vi "example-write-read-table.vi"() -> ()   [LabVIEW 2013]
uses:
  cfitsio-hdutypes.ctl
  gfitsio-write-column-u8-scalar.vi
  gfitsio-write-column-u8-1d.vi
  gfitsio-read-column-u8-scalar.vi
  gfitsio-read-column-u8-1d.vi
  gfitsio-write-column-i16-scalar.vi
  gfitsio-write-column-i16-1d.vi
  gfitsio-read-column-i16-scalar.vi
  gfitsio-read-column-i16-1d.vi
  gfitsio-write-column-i32-scalar.vi
  gfitsio-write-column-i32-1d.vi
  gfitsio-read-column-i32-scalar.vi
  gfitsio-read-column-i32-1d.vi
  gfitsio-write-column-sgl-scalar.vi
  gfitsio-write-column-sgl-1d.vi
  gfitsio-read-column-sgl-scalar.vi
  gfitsio-read-column-sgl-1d.vi
  gfitsio-write-column-dbl-scalar.vi
  gfitsio-write-column-dbl-1d.vi
  gfitsio-read-column-dbl-scalar.vi
  gfitsio-read-column-dbl-1d.vi
  gfitsio-write-column-boolean-scalar.vi
  gfitsio-write-column-boolean-1d.vi
  gfitsio-read-column-boolean-scalar.vi
  gfitsio-read-column-boolean-1d.vi
  gfitsio-write-column-csg-scalar.vi
  gfitsio-write-column-csg-1d.vi
  gfitsio-read-column-csg-scalar.vi
  gfitsio-read-column-csg-1d.vi
  gfitsio-write-column-cdb-scalar.vi
  gfitsio-write-column-cdb-1d.vi
  gfitsio-read-column-cdb-scalar.vi
  gfitsio-read-column-cdb-1d.vi
  gfitsio-write-column-string.vi
  gfitsio-read-column-string.vi
  gfitsio-write-column-datetime.vi
  gfitsio-read-column-datetime.vi
  gfitsio.lvlib
panel:
  out "error out":errorcluster
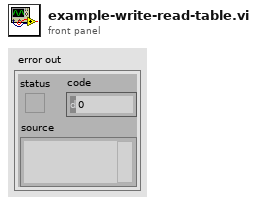
[diagram p1: front panel]
types:
  T1 = enum16{"open", "open or create", "create or replace", "create", "open (read only)"}
  T2 = typedef "gfitsio.lvlib/gfitsio-refnum.ctl" = refnum<k1>
  T3 = typedef "gfitsio.lvlib/cfitsio-hdutypes.ctl" = i32
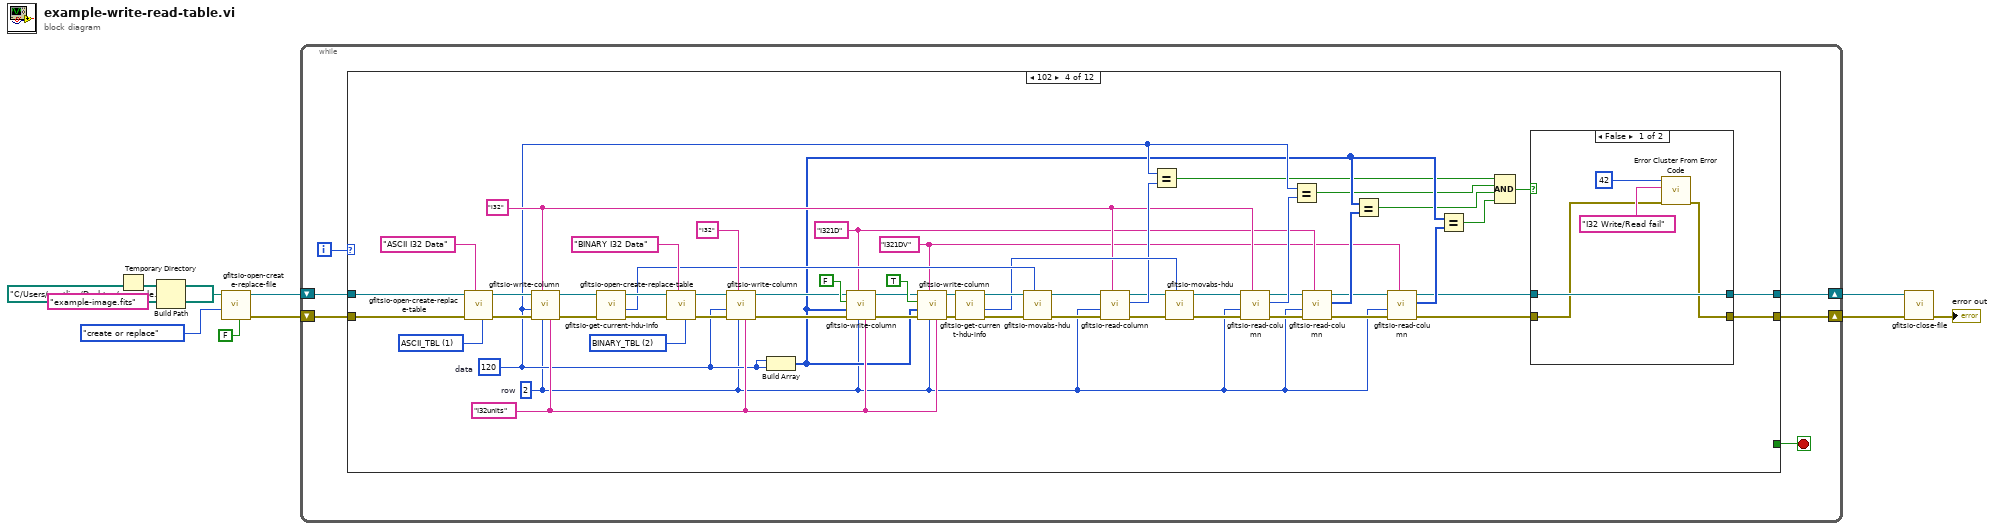
[diagram p0: block diagram]
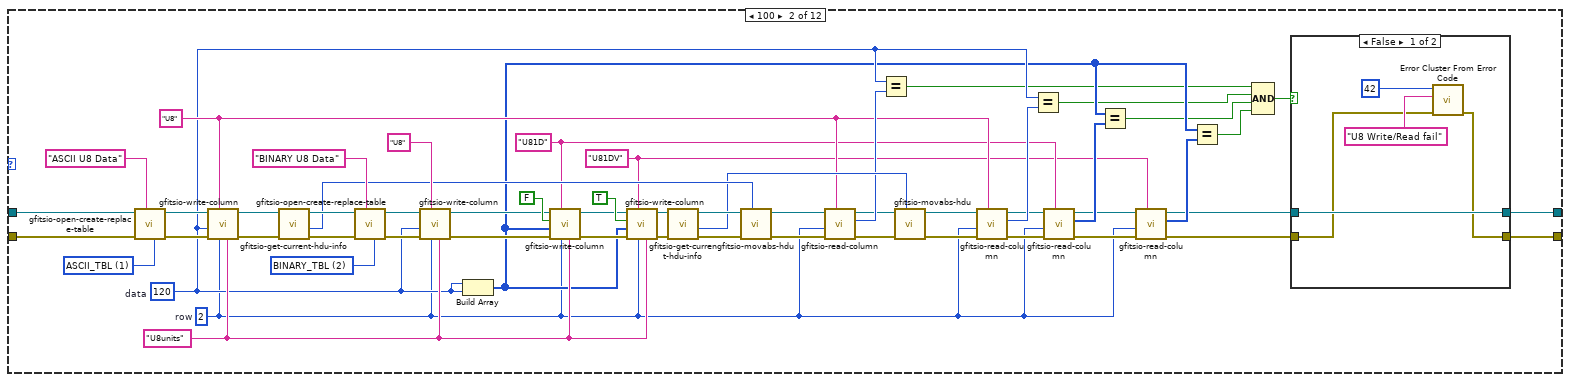
[diagram p3: hidden frame]
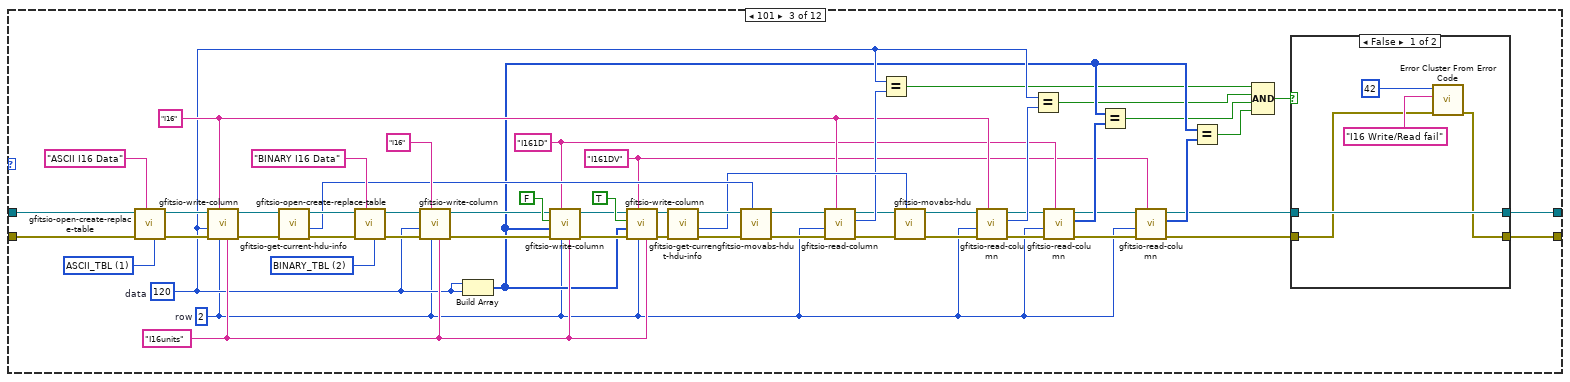
[diagram p5: hidden frame]
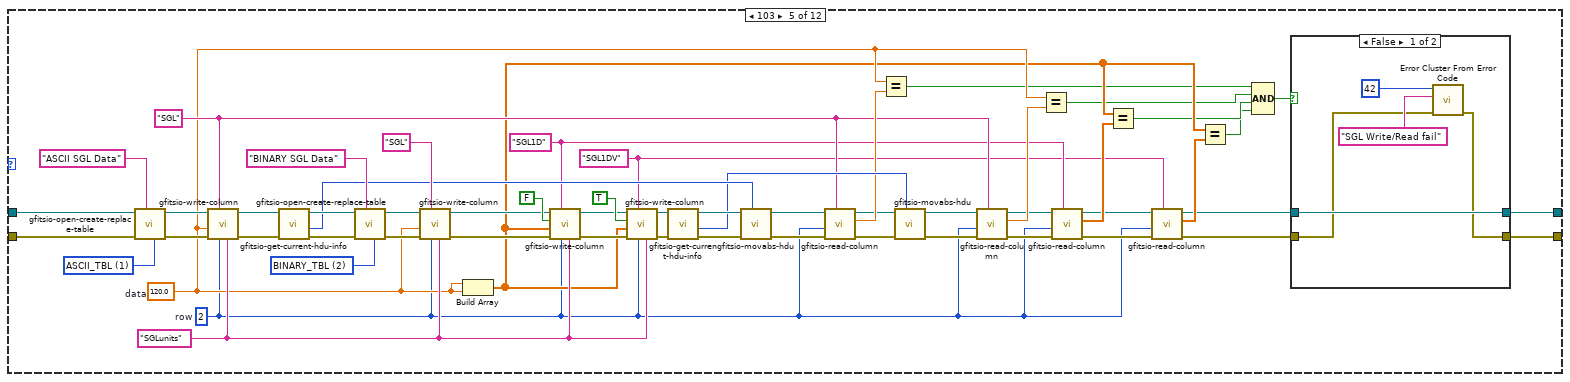
[diagram p8: hidden frame]
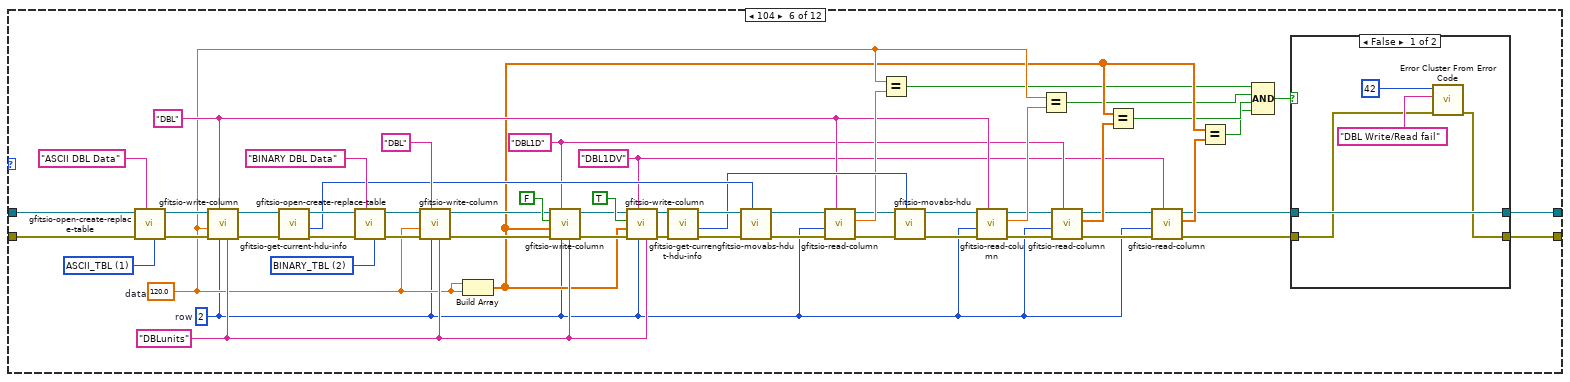
[diagram p10: hidden frame]
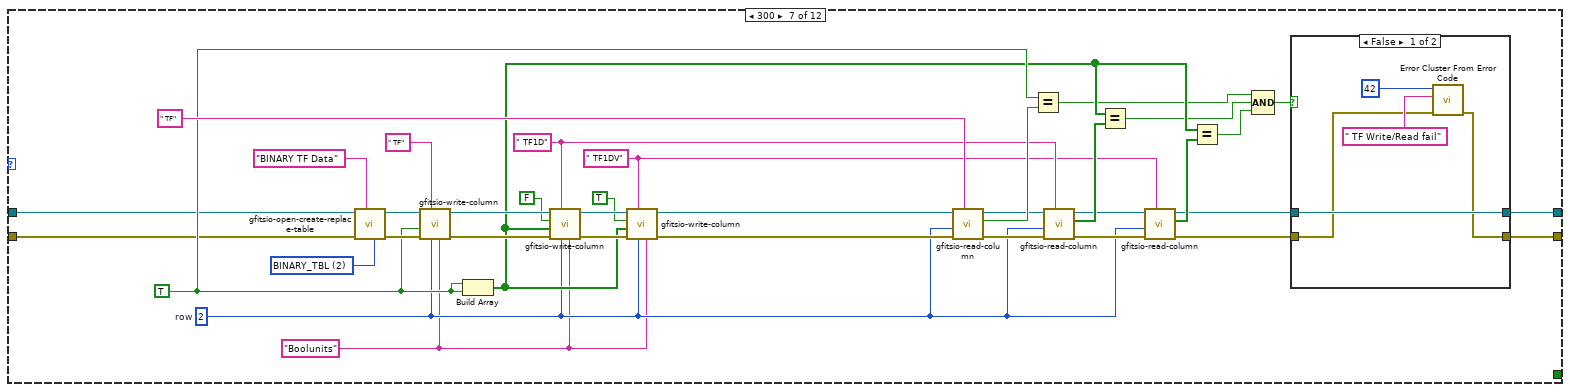
[diagram p12: hidden frame]
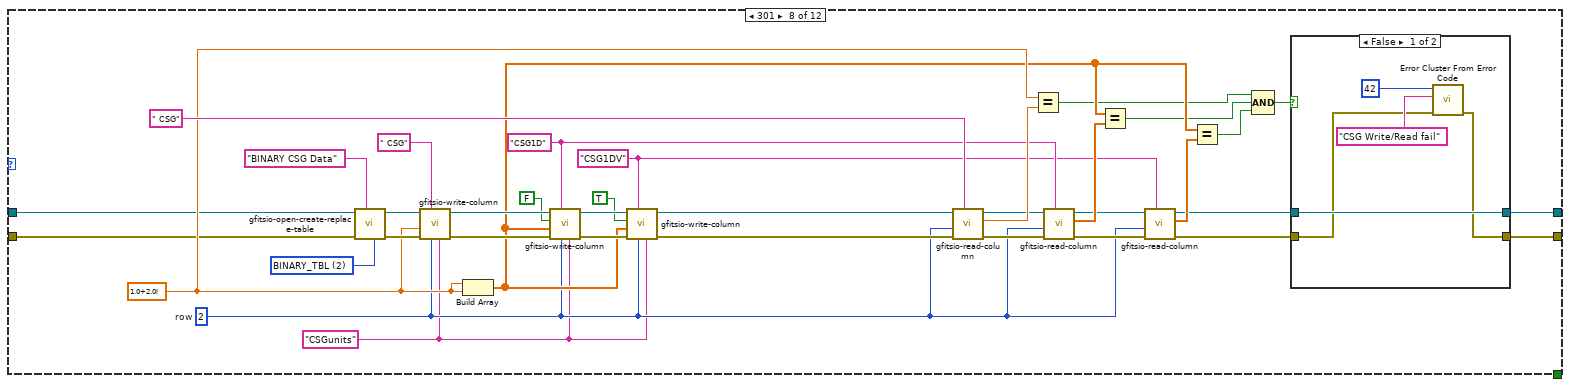
[diagram p14: hidden frame]
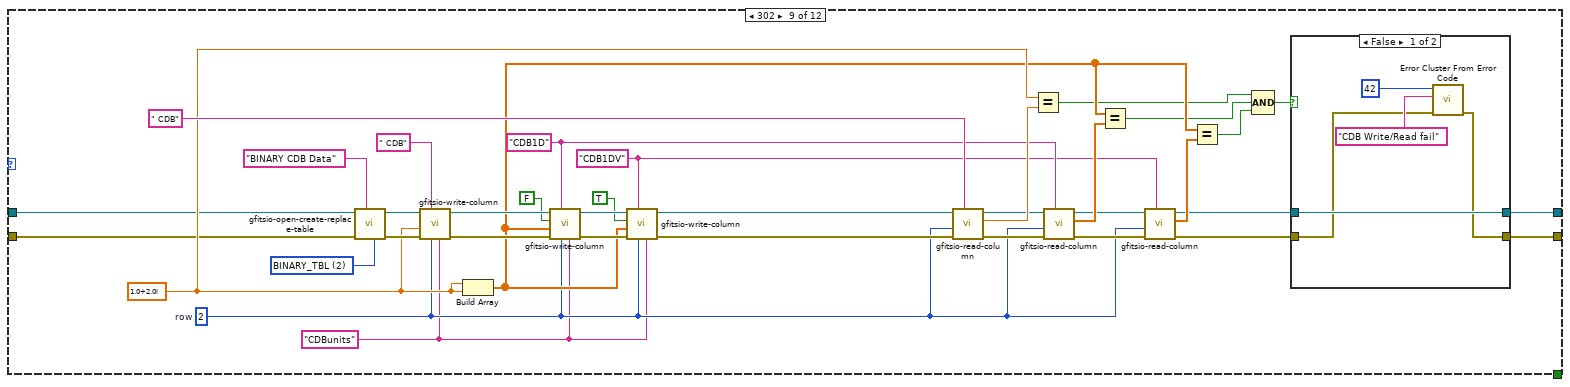
[diagram p16: hidden frame]
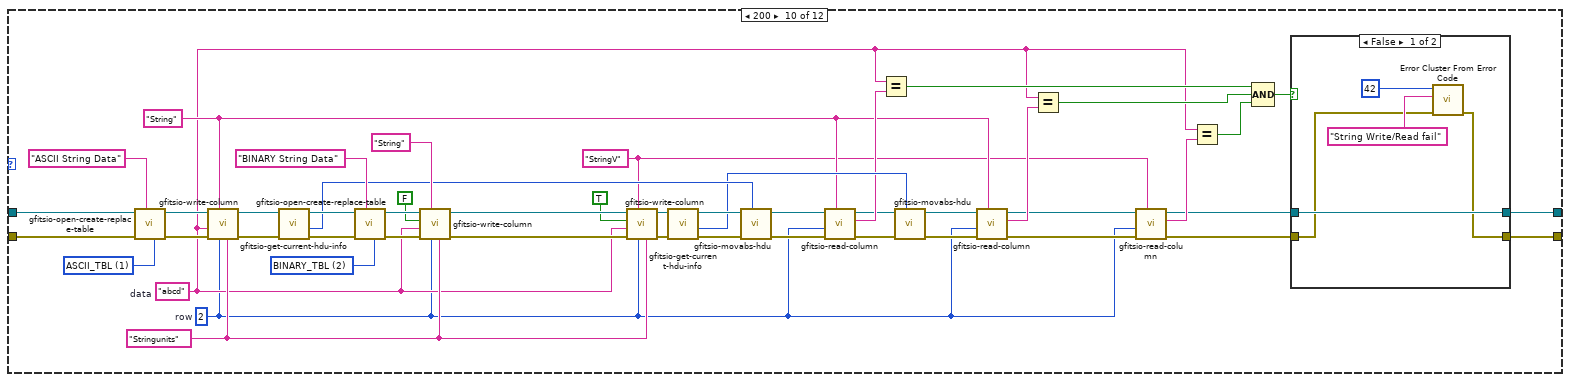
[diagram p18: hidden frame]
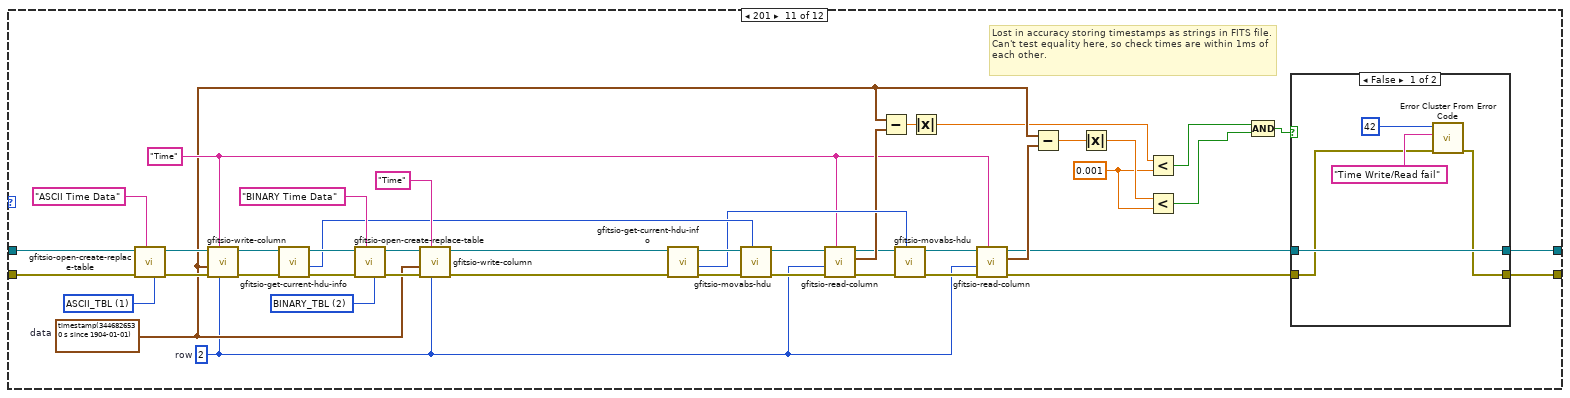
[diagram p20: hidden frame]
diagram:
  n1 = Temporary Directory() -> (w7:path)
  n2 = Build Path(base path=w7, name or relative path="example-image.fits") -> ()  [unwired: 1 out]
  n3 = call "gfitsio-open-create-replace-file.vi"("advisory dialog? (display:T)"=FALSE, "function (open)"=T1."create or replace", "file path (dialog if empty)"=path "C:/Users/ggatling/Desktop/example.fits") -> ("error out"=w9:errorcluster, "gfits refnum"=w10:T2)  [unwired: 6 in, 1 out]
  n4 = while {
    shift-right: [w14] -> w2
    shift-left: w10 -> [w16]
    shift-right: [w13] -> w1
    shift-left: w9 -> [w15]
    i -> [w12]
    stop <- w11 stop-if-true
    n5 = case shown="102" w12 {
      tunnel: w16 -> [w18 w75 w139 w203 w267 w331 w346 w390 w434 w519 w570 w580]
      tunnel: w15 -> [w17 w74 w138 w202 w266 w330 w345 w389 w433 w518 w569 w579]
      tunnel: [w18 w21 w85 w149 w213 w277 w348 w392 w436 w476 w539 w580] -> w14
      tunnel: [w17 w20 w84 w148 w212 w276 w347 w391 w435 w475 w538 w579] -> w13
      tunnel: [_ _ _ _ _ _ _ _ _ _ _ TRUE] -> w11
      frame Default {
      }
      frame 100 {
        w69 = T3 2 items=["ANY_HDU"=-1, "IMAGE_HDU"=0, "ASCII_TBL"=1, "BINARY_TBL"=2] ("table type (binary)")
        w33 = "U81DV" ("column")
        w34 = "U81D" ("column")
        w70 = T3 1 items=["ANY_HDU"=-1, "IMAGE_HDU"=0, "ASCII_TBL"=1, "BINARY_TBL"=2] ("table type (binary)")
        w58 = "U8units" ("units")
        w19 = 2  # row
        w30 = u8 120  # data
        w36 = "U8" ("column")
        n6 = call "gfitsio-open-create-replace-table.vi"("table type (binary)"=w70, "hdu name (dialog if empty)"="ASCII U8 Data", "error in (no error)"=w74, "gfits refnum"=w75) -> ("error out"=w72:errorcluster, "dup gfits refnum"=w73:T2)  [unwired: 5 in, 1 out]
        n7 = call-poly "gfitsio-write-column.vi"("units"=w58, "row"=w19, "column"=w36, "error in (no error)"=w72, "data"=w30, "gfits refnum"=w73) -> ("error out"=w56:errorcluster, "dup gfits refnum"=w57:T2)  [unwired: 4 in]
        n8 = call "gfitsio-get-current-hdu-info.vi"("error in (no error)"=w56, "gfits refnum"=w57) -> ("error out"=w51:errorcluster, "hdu number"=w49:i32, "dup gfits refnum"=w50:T2)  [unwired: 5 in, 2 out]
        n9 = call "gfitsio-open-create-replace-table.vi"("table type (binary)"=w69, "hdu name (dialog if empty)"="BINARY U8 Data", "error in (no error)"=w51, "gfits refnum"=w50) -> ("error out"=w60:errorcluster, "dup gfits refnum"=w59:T2)  [unwired: 5 in, 1 out]
        n10 = call-poly "gfitsio-write-column.vi"("units"=w58, "row"=w19, "column"="U8", "error in (no error)"=w60, "data"=w30, "gfits refnum"=w59) -> ("error out"=w64:errorcluster, "dup gfits refnum"=w63:T2)  [unwired: 4 in]
        n11 = Build Array(w30, w30) -> (w29:u8[])
        n12 = call-poly "gfitsio-write-column.vi"("units"=w58, "row"=w19, "column"=w34, "error in (no error)"=w64, "data"=w29, "variable length? (T:yes)"=FALSE, "gfits refnum"=w63) -> ("error out"=w66:errorcluster, "dup gfits refnum"=w65:T2)  [unwired: 3 in]
        n13 = call-poly "gfitsio-write-column.vi"("units"=w58, "row"=w19, "column"=w33, "error in (no error)"=w66, "data"=w29, "variable length? (T:yes)"=TRUE, "gfits refnum"=w65) -> ("error out"=w55:errorcluster, "dup gfits refnum"=w54:T2)  [unwired: 3 in]
        n14 = call "gfitsio-get-current-hdu-info.vi"("error in (no error)"=w55, "gfits refnum"=w54) -> ("error out"=w53:errorcluster, "hdu number"=w48:i32, "dup gfits refnum"=w52:T2)  [unwired: 5 in, 2 out]
        n15 = call "gfitsio-movabs-hdu.vi"("hdunum"=w49, "error in (no error)"=w53, "gfits refnum"=w52) -> ("error out"=w46:errorcluster, "dup gfits refnum"=w47:T2)  [unwired: 6 in, 1 out]
        n16 = call-poly "gfitsio-read-column.vi"("column"=w36, "error in (no error)"=w46, "row"=w19, "gfits refnum"=w47) -> ("error out"=w41:errorcluster, "data"=w45:u8, "dup gfits refnum"=w42:T2)  [unwired: 5 in]
        n17 = Equal?(x=w30, y=w45) -> (x = y?=w28:bool)
        n18 = call "gfitsio-movabs-hdu.vi"("hdunum"=w48, "error in (no error)"=w41, "gfits refnum"=w42) -> ("error out"=w39:errorcluster, "dup gfits refnum"=w40:T2)  [unwired: 6 in, 1 out]
        n19 = call-poly "gfitsio-read-column.vi"("column"=w36, "error in (no error)"=w39, "row"=w19, "gfits refnum"=w40) -> ("error out"=w37:errorcluster, "data"=w44:u8, "dup gfits refnum"=w38:T2)  [unwired: 5 in]
        n20 = Equal?(x=w30, y=w44) -> (x = y?=w27:bool)
        n21 = call-poly "gfitsio-read-column.vi"("column"=w34, "error in (no error)"=w37, "row"=w19, "gfits refnum"=w38) -> ("error out"=w31:errorcluster, "data"=w43:u8[], "dup gfits refnum"=w32:T2)  [unwired: 5 in]
        n22 = Equal?(x=w29, y=w43) -> (x = y?=w26:bool)
        n23 = call-poly "gfitsio-read-column.vi"("column"=w33, "error in (no error)"=w31, "row"=w19, "gfits refnum"=w32) -> ("error out"=w23:errorcluster, "data"=w35:u8[], "dup gfits refnum"=w24:T2)  [unwired: 5 in]
        n24 = Equal?(x=w29, y=w35) -> (x = y?=w25:bool)
        n25 = Compound Arithmetic op=AND(w28, w27, w26, w25) -> (w22:bool)
        n26 = case shown="False" w22 {
          tunnel: w24 -> [w80 w82]
          tunnel: w23 -> [w77 w81]
          tunnel: [w80 w82] -> w21
          tunnel: [w76 w81] -> w20
          frame False {
            n27 = call <vilib>:"Error Cluster From Error Code.vi"("error in (no error)"=w77, "error message (\"\")"="U8 Write/Read fail" ("error message (\"\")"), "error code (0)"=42) -> ("error out"=w76:errorcluster)  [unwired: 6 in]
          }
          frame True {
          }
        }
      }
      frame 101 {
        w133 = T3 2 items=["ANY_HDU"=-1, "IMAGE_HDU"=0, "ASCII_TBL"=1, "BINARY_TBL"=2] ("table type (binary)")
        w97 = "I161DV" ("column")
        w98 = "I161D" ("column")
        w134 = T3 1 items=["ANY_HDU"=-1, "IMAGE_HDU"=0, "ASCII_TBL"=1, "BINARY_TBL"=2] ("table type (binary)")
        w122 = "I16units" ("units")
        w83 = 2  # row
        w94 = i16 120  # data
        w100 = "I16" ("column")
        n28 = call "gfitsio-open-create-replace-table.vi"("table type (binary)"=w134, "hdu name (dialog if empty)"="ASCII I16 Data", "error in (no error)"=w138, "gfits refnum"=w139) -> ("error out"=w136:errorcluster, "dup gfits refnum"=w137:T2)  [unwired: 5 in, 1 out]
        n29 = call-poly "gfitsio-write-column.vi"("units"=w122, "row"=w83, "column"=w100, "error in (no error)"=w136, "data"=w94, "gfits refnum"=w137) -> ("error out"=w120:errorcluster, "dup gfits refnum"=w121:T2)  [unwired: 4 in]
        n30 = call "gfitsio-get-current-hdu-info.vi"("error in (no error)"=w120, "gfits refnum"=w121) -> ("error out"=w115:errorcluster, "hdu number"=w113:i32, "dup gfits refnum"=w114:T2)  [unwired: 5 in, 2 out]
        n31 = call "gfitsio-open-create-replace-table.vi"("table type (binary)"=w133, "hdu name (dialog if empty)"="BINARY I16 Data", "error in (no error)"=w115, "gfits refnum"=w114) -> ("error out"=w124:errorcluster, "dup gfits refnum"=w123:T2)  [unwired: 5 in, 1 out]
        n32 = call-poly "gfitsio-write-column.vi"("units"=w122, "row"=w83, "column"="I16", "error in (no error)"=w124, "data"=w94, "gfits refnum"=w123) -> ("error out"=w128:errorcluster, "dup gfits refnum"=w127:T2)  [unwired: 4 in]
        n33 = Build Array(w94, w94) -> (w93:i16[])
        n34 = call-poly "gfitsio-write-column.vi"("units"=w122, "row"=w83, "column"=w98, "error in (no error)"=w128, "data"=w93, "variable length? (T:yes)"=FALSE, "gfits refnum"=w127) -> ("error out"=w130:errorcluster, "dup gfits refnum"=w129:T2)  [unwired: 3 in]
        n35 = call-poly "gfitsio-write-column.vi"("units"=w122, "row"=w83, "column"=w97, "error in (no error)"=w130, "data"=w93, "variable length? (T:yes)"=TRUE, "gfits refnum"=w129) -> ("error out"=w119:errorcluster, "dup gfits refnum"=w118:T2)  [unwired: 3 in]
        n36 = call "gfitsio-get-current-hdu-info.vi"("error in (no error)"=w119, "gfits refnum"=w118) -> ("error out"=w117:errorcluster, "hdu number"=w112:i32, "dup gfits refnum"=w116:T2)  [unwired: 5 in, 2 out]
        n37 = call "gfitsio-movabs-hdu.vi"("hdunum"=w113, "error in (no error)"=w117, "gfits refnum"=w116) -> ("error out"=w110:errorcluster, "dup gfits refnum"=w111:T2)  [unwired: 6 in, 1 out]
        n38 = call-poly "gfitsio-read-column.vi"("column"=w100, "error in (no error)"=w110, "row"=w83, "gfits refnum"=w111) -> ("error out"=w105:errorcluster, "data"=w109:i16, "dup gfits refnum"=w106:T2)  [unwired: 5 in]
        n39 = Equal?(x=w94, y=w109) -> (x = y?=w92:bool)
        n40 = call "gfitsio-movabs-hdu.vi"("hdunum"=w112, "error in (no error)"=w105, "gfits refnum"=w106) -> ("error out"=w103:errorcluster, "dup gfits refnum"=w104:T2)  [unwired: 6 in, 1 out]
        n41 = call-poly "gfitsio-read-column.vi"("column"=w100, "error in (no error)"=w103, "row"=w83, "gfits refnum"=w104) -> ("error out"=w101:errorcluster, "data"=w108:i16, "dup gfits refnum"=w102:T2)  [unwired: 5 in]
        n42 = Equal?(x=w94, y=w108) -> (x = y?=w91:bool)
        n43 = call-poly "gfitsio-read-column.vi"("column"=w98, "error in (no error)"=w101, "row"=w83, "gfits refnum"=w102) -> ("error out"=w95:errorcluster, "data"=w107:i16[], "dup gfits refnum"=w96:T2)  [unwired: 5 in]
        n44 = Equal?(x=w93, y=w107) -> (x = y?=w90:bool)
        n45 = call-poly "gfitsio-read-column.vi"("column"=w97, "error in (no error)"=w95, "row"=w83, "gfits refnum"=w96) -> ("error out"=w87:errorcluster, "data"=w99:i16[], "dup gfits refnum"=w88:T2)  [unwired: 5 in]
        n46 = Equal?(x=w93, y=w99) -> (x = y?=w89:bool)
        n47 = Compound Arithmetic op=AND(w92, w91, w90, w89) -> (w86:bool)
        n48 = case shown="False" w86 {
          tunnel: w88 -> [w144 w146]
          tunnel: w87 -> [w141 w145]
          tunnel: [w144 w146] -> w85
          tunnel: [w140 w145] -> w84
          frame False {
            n49 = call <vilib>:"Error Cluster From Error Code.vi"("error in (no error)"=w141, "error message (\"\")"="I16 Write/Read fail" ("error message (\"\")"), "error code (0)"=42) -> ("error out"=w140:errorcluster)  [unwired: 6 in]
          }
          frame True {
          }
        }
      }
      frame 102 {
        w197 = T3 2 items=["ANY_HDU"=-1, "IMAGE_HDU"=0, "ASCII_TBL"=1, "BINARY_TBL"=2] ("table type (binary)")
        w161 = "I321DV" ("column")
        w162 = "I321D" ("column")
        w198 = T3 1 items=["ANY_HDU"=-1, "IMAGE_HDU"=0, "ASCII_TBL"=1, "BINARY_TBL"=2] ("table type (binary)")
        w186 = "I32units" ("units")
        w147 = 2  # row
        w158 = 120  # data
        w164 = "I32" ("column")
        n50 = call "gfitsio-open-create-replace-table.vi"("table type (binary)"=w198, "hdu name (dialog if empty)"="ASCII I32 Data", "error in (no error)"=w202, "gfits refnum"=w203) -> ("error out"=w200:errorcluster, "dup gfits refnum"=w201:T2)  [unwired: 5 in, 1 out]
        n51 = call-poly "gfitsio-write-column.vi"("units"=w186, "row"=w147, "column"=w164, "error in (no error)"=w200, "data"=w158, "gfits refnum"=w201) -> ("error out"=w184:errorcluster, "dup gfits refnum"=w185:T2)  [unwired: 4 in]
        n52 = call "gfitsio-get-current-hdu-info.vi"("error in (no error)"=w184, "gfits refnum"=w185) -> ("error out"=w179:errorcluster, "hdu number"=w177:i32, "dup gfits refnum"=w178:T2)  [unwired: 5 in, 2 out]
        n53 = call "gfitsio-open-create-replace-table.vi"("table type (binary)"=w197, "hdu name (dialog if empty)"="BINARY I32 Data", "error in (no error)"=w179, "gfits refnum"=w178) -> ("error out"=w188:errorcluster, "dup gfits refnum"=w187:T2)  [unwired: 5 in, 1 out]
        n54 = call-poly "gfitsio-write-column.vi"("units"=w186, "row"=w147, "column"="I32", "error in (no error)"=w188, "data"=w158, "gfits refnum"=w187) -> ("error out"=w192:errorcluster, "dup gfits refnum"=w191:T2)  [unwired: 4 in]
        n55 = Build Array(w158, w158) -> (w157:i32[])
        n56 = call-poly "gfitsio-write-column.vi"("units"=w186, "row"=w147, "column"=w162, "error in (no error)"=w192, "data"=w157, "variable length? (T:yes)"=FALSE, "gfits refnum"=w191) -> ("error out"=w194:errorcluster, "dup gfits refnum"=w193:T2)  [unwired: 3 in]
        n57 = call-poly "gfitsio-write-column.vi"("units"=w186, "row"=w147, "column"=w161, "error in (no error)"=w194, "data"=w157, "variable length? (T:yes)"=TRUE, "gfits refnum"=w193) -> ("error out"=w183:errorcluster, "dup gfits refnum"=w182:T2)  [unwired: 3 in]
        n58 = call "gfitsio-get-current-hdu-info.vi"("error in (no error)"=w183, "gfits refnum"=w182) -> ("error out"=w181:errorcluster, "hdu number"=w176:i32, "dup gfits refnum"=w180:T2)  [unwired: 5 in, 2 out]
        n59 = call "gfitsio-movabs-hdu.vi"("hdunum"=w177, "error in (no error)"=w181, "gfits refnum"=w180) -> ("error out"=w174:errorcluster, "dup gfits refnum"=w175:T2)  [unwired: 6 in, 1 out]
        n60 = call-poly "gfitsio-read-column.vi"("column"=w164, "error in (no error)"=w174, "row"=w147, "gfits refnum"=w175) -> ("error out"=w169:errorcluster, "data"=w173:i32, "dup gfits refnum"=w170:T2)  [unwired: 5 in]
        n61 = Equal?(x=w158, y=w173) -> (x = y?=w156:bool)
        n62 = call "gfitsio-movabs-hdu.vi"("hdunum"=w176, "error in (no error)"=w169, "gfits refnum"=w170) -> ("error out"=w167:errorcluster, "dup gfits refnum"=w168:T2)  [unwired: 6 in, 1 out]
        n63 = call-poly "gfitsio-read-column.vi"("column"=w164, "error in (no error)"=w167, "row"=w147, "gfits refnum"=w168) -> ("error out"=w165:errorcluster, "data"=w172:i32, "dup gfits refnum"=w166:T2)  [unwired: 5 in]
        n64 = Equal?(x=w158, y=w172) -> (x = y?=w155:bool)
        n65 = call-poly "gfitsio-read-column.vi"("column"=w162, "error in (no error)"=w165, "row"=w147, "gfits refnum"=w166) -> ("error out"=w159:errorcluster, "data"=w171:i32[], "dup gfits refnum"=w160:T2)  [unwired: 5 in]
        n66 = Equal?(x=w157, y=w171) -> (x = y?=w154:bool)
        n67 = call-poly "gfitsio-read-column.vi"("column"=w161, "error in (no error)"=w159, "row"=w147, "gfits refnum"=w160) -> ("error out"=w151:errorcluster, "data"=w163:i32[], "dup gfits refnum"=w152:T2)  [unwired: 5 in]
        n68 = Equal?(x=w157, y=w163) -> (x = y?=w153:bool)
        n69 = Compound Arithmetic op=AND(w156, w155, w154, w153) -> (w150:bool)
        n70 = case shown="False" w150 {
          tunnel: w152 -> [w208 w210]
          tunnel: w151 -> [w205 w209]
          tunnel: [w208 w210] -> w149
          tunnel: [w204 w209] -> w148
          frame False {
            n71 = call <vilib>:"Error Cluster From Error Code.vi"("error in (no error)"=w205, "error message (\"\")"="I32 Write/Read fail" ("error message (\"\")"), "error code (0)"=42) -> ("error out"=w204:errorcluster)  [unwired: 6 in]
          }
          frame True {
          }
        }
      }
      frame 103 {
        w261 = T3 2 items=["ANY_HDU"=-1, "IMAGE_HDU"=0, "ASCII_TBL"=1, "BINARY_TBL"=2] ("table type (binary)")
        w225 = "SGL1DV" ("column")
        w226 = "SGL1D" ("column")
        w262 = T3 1 items=["ANY_HDU"=-1, "IMAGE_HDU"=0, "ASCII_TBL"=1, "BINARY_TBL"=2] ("table type (binary)")
        w250 = "SGLunits" ("units")
        w211 = 2  # row
        w222 = sgl 120.0  # data
        w228 = "SGL" ("column")
        n72 = call "gfitsio-open-create-replace-table.vi"("table type (binary)"=w262, "hdu name (dialog if empty)"="ASCII SGL Data", "error in (no error)"=w266, "gfits refnum"=w267) -> ("error out"=w264:errorcluster, "dup gfits refnum"=w265:T2)  [unwired: 5 in, 1 out]
        n73 = call-poly "gfitsio-write-column.vi"("units"=w250, "row"=w211, "column"=w228, "error in (no error)"=w264, "data"=w222, "gfits refnum"=w265) -> ("error out"=w248:errorcluster, "dup gfits refnum"=w249:T2)  [unwired: 4 in]
        n74 = call "gfitsio-get-current-hdu-info.vi"("error in (no error)"=w248, "gfits refnum"=w249) -> ("error out"=w243:errorcluster, "hdu number"=w241:i32, "dup gfits refnum"=w242:T2)  [unwired: 5 in, 2 out]
        n75 = call "gfitsio-open-create-replace-table.vi"("table type (binary)"=w261, "hdu name (dialog if empty)"="BINARY SGL Data", "error in (no error)"=w243, "gfits refnum"=w242) -> ("error out"=w252:errorcluster, "dup gfits refnum"=w251:T2)  [unwired: 5 in, 1 out]
        n76 = call-poly "gfitsio-write-column.vi"("units"=w250, "row"=w211, "column"="SGL", "error in (no error)"=w252, "data"=w222, "gfits refnum"=w251) -> ("error out"=w256:errorcluster, "dup gfits refnum"=w255:T2)  [unwired: 4 in]
        n77 = Build Array(w222, w222) -> (w221:sgl[])
        n78 = call-poly "gfitsio-write-column.vi"("units"=w250, "row"=w211, "column"=w226, "error in (no error)"=w256, "data"=w221, "variable length? (T:yes)"=FALSE, "gfits refnum"=w255) -> ("error out"=w258:errorcluster, "dup gfits refnum"=w257:T2)  [unwired: 3 in]
        n79 = call-poly "gfitsio-write-column.vi"("units"=w250, "row"=w211, "column"=w225, "error in (no error)"=w258, "data"=w221, "variable length? (T:yes)"=TRUE, "gfits refnum"=w257) -> ("error out"=w247:errorcluster, "dup gfits refnum"=w246:T2)  [unwired: 3 in]
        n80 = call "gfitsio-get-current-hdu-info.vi"("error in (no error)"=w247, "gfits refnum"=w246) -> ("error out"=w245:errorcluster, "hdu number"=w240:i32, "dup gfits refnum"=w244:T2)  [unwired: 5 in, 2 out]
        n81 = call "gfitsio-movabs-hdu.vi"("hdunum"=w241, "error in (no error)"=w245, "gfits refnum"=w244) -> ("error out"=w238:errorcluster, "dup gfits refnum"=w239:T2)  [unwired: 6 in, 1 out]
        n82 = call-poly "gfitsio-read-column.vi"("column"=w228, "error in (no error)"=w238, "row"=w211, "gfits refnum"=w239) -> ("error out"=w233:errorcluster, "data"=w237:sgl, "dup gfits refnum"=w234:T2)  [unwired: 5 in]
        n83 = Equal?(x=w222, y=w237) -> (x = y?=w220:bool)
        n84 = call "gfitsio-movabs-hdu.vi"("hdunum"=w240, "error in (no error)"=w233, "gfits refnum"=w234) -> ("error out"=w231:errorcluster, "dup gfits refnum"=w232:T2)  [unwired: 6 in, 1 out]
        n85 = call-poly "gfitsio-read-column.vi"("column"=w228, "error in (no error)"=w231, "row"=w211, "gfits refnum"=w232) -> ("error out"=w229:errorcluster, "data"=w236:sgl, "dup gfits refnum"=w230:T2)  [unwired: 5 in]
        n86 = Equal?(x=w222, y=w236) -> (x = y?=w219:bool)
        n87 = call-poly "gfitsio-read-column.vi"("column"=w226, "error in (no error)"=w229, "row"=w211, "gfits refnum"=w230) -> ("error out"=w223:errorcluster, "data"=w235:sgl[], "dup gfits refnum"=w224:T2)  [unwired: 5 in]
        n88 = Equal?(x=w221, y=w235) -> (x = y?=w218:bool)
        n89 = call-poly "gfitsio-read-column.vi"("column"=w225, "error in (no error)"=w223, "row"=w211, "gfits refnum"=w224) -> ("error out"=w215:errorcluster, "data"=w227:sgl[], "dup gfits refnum"=w216:T2)  [unwired: 5 in]
        n90 = Equal?(x=w221, y=w227) -> (x = y?=w217:bool)
        n91 = Compound Arithmetic op=AND(w220, w219, w218, w217) -> (w214:bool)
        n92 = case shown="False" w214 {
          tunnel: w216 -> [w272 w274]
          tunnel: w215 -> [w269 w273]
          tunnel: [w272 w274] -> w213
          tunnel: [w268 w273] -> w212
          frame False {
            n93 = call <vilib>:"Error Cluster From Error Code.vi"("error in (no error)"=w269, "error message (\"\")"="SGL Write/Read fail" ("error message (\"\")"), "error code (0)"=42) -> ("error out"=w268:errorcluster)  [unwired: 6 in]
          }
          frame True {
          }
        }
      }
      frame 104 {
        w325 = T3 2 items=["ANY_HDU"=-1, "IMAGE_HDU"=0, "ASCII_TBL"=1, "BINARY_TBL"=2] ("table type (binary)")
        w289 = "DBL1DV" ("column")
        w290 = "DBL1D" ("column")
        w326 = T3 1 items=["ANY_HDU"=-1, "IMAGE_HDU"=0, "ASCII_TBL"=1, "BINARY_TBL"=2] ("table type (binary)")
        w314 = "DBLunits" ("units")
        w275 = 2  # row
        w286 = 120.0  # data
        w292 = "DBL" ("column")
        n94 = call "gfitsio-open-create-replace-table.vi"("table type (binary)"=w326, "hdu name (dialog if empty)"="ASCII DBL Data", "error in (no error)"=w330, "gfits refnum"=w331) -> ("error out"=w328:errorcluster, "dup gfits refnum"=w329:T2)  [unwired: 5 in, 1 out]
        n95 = call-poly "gfitsio-write-column.vi"("units"=w314, "row"=w275, "column"=w292, "error in (no error)"=w328, "data"=w286, "gfits refnum"=w329) -> ("error out"=w312:errorcluster, "dup gfits refnum"=w313:T2)  [unwired: 4 in]
        n96 = call "gfitsio-get-current-hdu-info.vi"("error in (no error)"=w312, "gfits refnum"=w313) -> ("error out"=w307:errorcluster, "hdu number"=w305:i32, "dup gfits refnum"=w306:T2)  [unwired: 5 in, 2 out]
        n97 = call "gfitsio-open-create-replace-table.vi"("table type (binary)"=w325, "hdu name (dialog if empty)"="BINARY DBL Data", "error in (no error)"=w307, "gfits refnum"=w306) -> ("error out"=w316:errorcluster, "dup gfits refnum"=w315:T2)  [unwired: 5 in, 1 out]
        n98 = call-poly "gfitsio-write-column.vi"("units"=w314, "row"=w275, "column"="DBL", "error in (no error)"=w316, "data"=w286, "gfits refnum"=w315) -> ("error out"=w320:errorcluster, "dup gfits refnum"=w319:T2)  [unwired: 4 in]
        n99 = Build Array(w286, w286) -> (w285:dbl[])
        n100 = call-poly "gfitsio-write-column.vi"("units"=w314, "row"=w275, "column"=w290, "error in (no error)"=w320, "data"=w285, "variable length? (T:yes)"=FALSE, "gfits refnum"=w319) -> ("error out"=w322:errorcluster, "dup gfits refnum"=w321:T2)  [unwired: 3 in]
        n101 = call-poly "gfitsio-write-column.vi"("units"=w314, "row"=w275, "column"=w289, "error in (no error)"=w322, "data"=w285, "variable length? (T:yes)"=TRUE, "gfits refnum"=w321) -> ("error out"=w311:errorcluster, "dup gfits refnum"=w310:T2)  [unwired: 3 in]
        n102 = call "gfitsio-get-current-hdu-info.vi"("error in (no error)"=w311, "gfits refnum"=w310) -> ("error out"=w309:errorcluster, "hdu number"=w304:i32, "dup gfits refnum"=w308:T2)  [unwired: 5 in, 2 out]
        n103 = call "gfitsio-movabs-hdu.vi"("hdunum"=w305, "error in (no error)"=w309, "gfits refnum"=w308) -> ("error out"=w302:errorcluster, "dup gfits refnum"=w303:T2)  [unwired: 6 in, 1 out]
        n104 = call-poly "gfitsio-read-column.vi"("column"=w292, "error in (no error)"=w302, "row"=w275, "gfits refnum"=w303) -> ("error out"=w297:errorcluster, "data"=w301:dbl, "dup gfits refnum"=w298:T2)  [unwired: 5 in]
        n105 = Equal?(x=w286, y=w301) -> (x = y?=w284:bool)
        n106 = call "gfitsio-movabs-hdu.vi"("hdunum"=w304, "error in (no error)"=w297, "gfits refnum"=w298) -> ("error out"=w295:errorcluster, "dup gfits refnum"=w296:T2)  [unwired: 6 in, 1 out]
        n107 = call-poly "gfitsio-read-column.vi"("column"=w292, "error in (no error)"=w295, "row"=w275, "gfits refnum"=w296) -> ("error out"=w293:errorcluster, "data"=w300:dbl, "dup gfits refnum"=w294:T2)  [unwired: 5 in]
        n108 = Equal?(x=w286, y=w300) -> (x = y?=w283:bool)
        n109 = call-poly "gfitsio-read-column.vi"("column"=w290, "error in (no error)"=w293, "row"=w275, "gfits refnum"=w294) -> ("error out"=w287:errorcluster, "data"=w299:dbl[], "dup gfits refnum"=w288:T2)  [unwired: 5 in]
        n110 = Equal?(x=w285, y=w299) -> (x = y?=w282:bool)
        n111 = call-poly "gfitsio-read-column.vi"("column"=w289, "error in (no error)"=w287, "row"=w275, "gfits refnum"=w288) -> ("error out"=w279:errorcluster, "data"=w291:dbl[], "dup gfits refnum"=w280:T2)  [unwired: 5 in]
        n112 = Equal?(x=w285, y=w291) -> (x = y?=w281:bool)
        n113 = Compound Arithmetic op=AND(w284, w283, w282, w281) -> (w278:bool)
        n114 = case shown="False" w278 {
          tunnel: w280 -> [w336 w338]
          tunnel: w279 -> [w333 w337]
          tunnel: [w336 w338] -> w277
          tunnel: [w332 w337] -> w276
          frame False {
            n115 = call <vilib>:"Error Cluster From Error Code.vi"("error in (no error)"=w333, "error message (\"\")"="DBL Write/Read fail" ("error message (\"\")"), "error code (0)"=42) -> ("error out"=w332:errorcluster)  [unwired: 6 in]
          }
          frame True {
          }
        }
      }
      frame 300 {
        w339 = "Boolunits" ("column")
        w375 = T3 2 items=["ANY_HDU"=-1, "IMAGE_HDU"=0, "ASCII_TBL"=1, "BINARY_TBL"=2] ("table type (binary)")
        w359 = " TF1DV" ("column")
        w360 = " TF1D" ("column")
        w340 = 2  # row
        w356 = TRUE
        n116 = call "gfitsio-open-create-replace-table.vi"("table type (binary)"=w375, "hdu name (dialog if empty)"="BINARY TF Data", "error in (no error)"=w345, "gfits refnum"=w346) -> ("error out"=w368:errorcluster, "dup gfits refnum"=w367:T2)  [unwired: 5 in, 1 out]
        n117 = call-poly "gfitsio-write-column.vi"("units"=w339, "row"=w340, "column"=" TF", "error in (no error)"=w368, "data"=w356, "gfits refnum"=w367) -> ("error out"=w372:errorcluster, "dup gfits refnum"=w371:T2)  [unwired: 4 in]
        n118 = Build Array(w356, w356) -> (w355:bool[])
        n119 = call-poly "gfitsio-write-column.vi"("units"=w339, "row"=w340, "column"=w360, "error in (no error)"=w372, "data"=w355, "Variable Size? (F)"=FALSE ("variable length? (T:yes)"), "gfits refnum"=w371) -> ("error out"=w374:errorcluster, "dup gfits refnum"=w373:T2)  [unwired: 3 in]
        n120 = call-poly "gfitsio-write-column.vi"("units"=w339, "row"=w340, "column"=w359, "error in (no error)"=w374, "data"=w355, "Variable Size? (F)"=TRUE ("variable length? (T:yes)"), "gfits refnum"=w373) -> ("error out"=w343:errorcluster, "dup gfits refnum"=w344:T2)  [unwired: 3 in]
        n121 = call-poly "gfitsio-read-column.vi"("column"=" TF", "error in (no error)"=w343, "row"=w340, "gfits refnum"=w344) -> ("error out"=w363:errorcluster, "data"=w366:bool, "dup gfits refnum"=w364:T2)  [unwired: 5 in]
        n122 = Equal?(x=w356, y=w366) -> (x = y?=w354:bool)
        n123 = call-poly "gfitsio-read-column.vi"("column"=w360, "error in (no error)"=w363, "row"=w340, "gfits refnum"=w364) -> ("error out"=w357:errorcluster, "data"=w365:bool[], "dup gfits refnum"=w358:T2)  [unwired: 5 in]
        n124 = Equal?(x=w355, y=w365) -> (x = y?=w353:bool)
        n125 = call-poly "gfitsio-read-column.vi"("column"=w359, "error in (no error)"=w357, "row"=w340, "gfits refnum"=w358) -> ("error out"=w350:errorcluster, "data"=w361:bool[], "dup gfits refnum"=w351:T2)  [unwired: 5 in]
        n126 = Equal?(x=w355, y=w361) -> (x = y?=w352:bool)
        n127 = Compound Arithmetic op=AND(w354, w353, w352) -> (w349:bool)
        n128 = case shown="False" w349 {
          tunnel: w351 -> [w380 w382]
          tunnel: w350 -> [w377 w381]
          tunnel: [w380 w382] -> w348
          tunnel: [w376 w381] -> w347
          frame False {
            n129 = call <vilib>:"Error Cluster From Error Code.vi"("error in (no error)"=w377, "error message (\"\")"=" TF Write/Read fail" ("error message (\"\")"), "error code (0)"=42) -> ("error out"=w376:errorcluster)  [unwired: 6 in]
          }
          frame True {
          }
        }
      }
      frame 301 {
        w383 = "CSGunits" ("units")
        w419 = T3 2 items=["ANY_HDU"=-1, "IMAGE_HDU"=0, "ASCII_TBL"=1, "BINARY_TBL"=2] ("table type (binary)")
        w403 = "CSG1DV" ("column")
        w404 = "CSG1D" ("column")
        w384 = 2  # row
        w400 = csg 1.0+2.0i
        n130 = call "gfitsio-open-create-replace-table.vi"("table type (binary)"=w419, "hdu name (dialog if empty)"="BINARY CSG Data", "error in (no error)"=w389, "gfits refnum"=w390) -> ("error out"=w412:errorcluster, "dup gfits refnum"=w411:T2)  [unwired: 5 in, 1 out]
        n131 = call-poly "gfitsio-write-column.vi"("units"=w383, "row"=w384, "column"=" CSG", "error in (no error)"=w412, "data"=w400, "gfits refnum"=w411) -> ("error out"=w416:errorcluster, "dup gfits refnum"=w415:T2)  [unwired: 4 in]
        n132 = Build Array(w400, w400) -> (w399:csg[])
        n133 = call-poly "gfitsio-write-column.vi"("units"=w383, "row"=w384, "column"=w404, "error in (no error)"=w416, "data"=w399, "variable length? (T:yes)"=FALSE, "gfits refnum"=w415) -> ("error out"=w418:errorcluster, "dup gfits refnum"=w417:T2)  [unwired: 3 in]
        n134 = call-poly "gfitsio-write-column.vi"("units"=w383, "row"=w384, "column"=w403, "error in (no error)"=w418, "data"=w399, "variable length? (T:yes)"=TRUE, "gfits refnum"=w417) -> ("error out"=w387:errorcluster, "dup gfits refnum"=w388:T2)  [unwired: 3 in]
        n135 = call-poly "gfitsio-read-column.vi"("column"=" CSG", "error in (no error)"=w387, "row"=w384, "gfits refnum"=w388) -> ("error out"=w407:errorcluster, "data"=w410:csg, "dup gfits refnum"=w408:T2)  [unwired: 5 in]
        n136 = Equal?(x=w400, y=w410) -> (x = y?=w398:bool)
        n137 = call-poly "gfitsio-read-column.vi"("column"=w404, "error in (no error)"=w407, "row"=w384, "gfits refnum"=w408) -> ("error out"=w401:errorcluster, "data"=w409:csg[], "dup gfits refnum"=w402:T2)  [unwired: 5 in]
        n138 = Equal?(x=w399, y=w409) -> (x = y?=w397:bool)
        n139 = call-poly "gfitsio-read-column.vi"("column"=w403, "error in (no error)"=w401, "row"=w384, "gfits refnum"=w402) -> ("error out"=w394:errorcluster, "data"=w405:csg[], "dup gfits refnum"=w395:T2)  [unwired: 5 in]
        n140 = Equal?(x=w399, y=w405) -> (x = y?=w396:bool)
        n141 = Compound Arithmetic op=AND(w398, w397, w396) -> (w393:bool)
        n142 = case shown="False" w393 {
          tunnel: w395 -> [w424 w426]
          tunnel: w394 -> [w421 w425]
          tunnel: [w424 w426] -> w392
          tunnel: [w420 w425] -> w391
          frame False {
            n143 = call <vilib>:"Error Cluster From Error Code.vi"("error in (no error)"=w421, "error message (\"\")"="CSG Write/Read fail" ("error message (\"\")"), "error code (0)"=42) -> ("error out"=w420:errorcluster)  [unwired: 6 in]
          }
          frame True {
          }
        }
      }
      frame 302 {
        w427 = "CDBunits" ("units")
        w463 = T3 2 items=["ANY_HDU"=-1, "IMAGE_HDU"=0, "ASCII_TBL"=1, "BINARY_TBL"=2] ("table type (binary)")
        w447 = "CDB1DV" ("column")
        w448 = "CDB1D" ("column")
        w428 = 2  # row
        w444 = cdb 1.0+2.0i
        n144 = call "gfitsio-open-create-replace-table.vi"("table type (binary)"=w463, "hdu name (dialog if empty)"="BINARY CDB Data", "error in (no error)"=w433, "gfits refnum"=w434) -> ("error out"=w456:errorcluster, "dup gfits refnum"=w455:T2)  [unwired: 5 in, 1 out]
        n145 = call-poly "gfitsio-write-column.vi"("units"=w427, "row"=w428, "column"=" CDB", "error in (no error)"=w456, "data"=w444, "gfits refnum"=w455) -> ("error out"=w460:errorcluster, "dup gfits refnum"=w459:T2)  [unwired: 4 in]
        n146 = Build Array(w444, w444) -> (w443:cdb[])
        n147 = call-poly "gfitsio-write-column.vi"("units"=w427, "row"=w428, "column"=w448, "error in (no error)"=w460, "data"=w443, "variable length? (T:yes)"=FALSE, "gfits refnum"=w459) -> ("error out"=w462:errorcluster, "dup gfits refnum"=w461:T2)  [unwired: 3 in]
        n148 = call-poly "gfitsio-write-column.vi"("units"=w427, "row"=w428, "column"=w447, "error in (no error)"=w462, "data"=w443, "variable length? (T:yes)"=TRUE, "gfits refnum"=w461) -> ("error out"=w431:errorcluster, "dup gfits refnum"=w432:T2)  [unwired: 3 in]
        n149 = call-poly "gfitsio-read-column.vi"("column"=" CDB", "error in (no error)"=w431, "row"=w428, "gfits refnum"=w432) -> ("error out"=w451:errorcluster, "data"=w454:cdb, "dup gfits refnum"=w452:T2)  [unwired: 5 in]
        n150 = Equal?(x=w444, y=w454) -> (x = y?=w442:bool)
        n151 = call-poly "gfitsio-read-column.vi"("column"=w448, "error in (no error)"=w451, "row"=w428, "gfits refnum"=w452) -> ("error out"=w445:errorcluster, "data"=w453:cdb[], "dup gfits refnum"=w446:T2)  [unwired: 5 in]
        n152 = Equal?(x=w443, y=w453) -> (x = y?=w441:bool)
        n153 = call-poly "gfitsio-read-column.vi"("column"=w447, "error in (no error)"=w445, "row"=w428, "gfits refnum"=w446) -> ("error out"=w438:errorcluster, "data"=w449:cdb[], "dup gfits refnum"=w439:T2)  [unwired: 5 in]
        n154 = Equal?(x=w443, y=w449) -> (x = y?=w440:bool)
        n155 = Compound Arithmetic op=AND(w442, w441, w440) -> (w437:bool)
        n156 = case shown="False" w437 {
          tunnel: w439 -> [w468 w470]
          tunnel: w438 -> [w465 w469]
          tunnel: [w468 w470] -> w436
          tunnel: [w464 w469] -> w435
          frame False {
            n157 = call <vilib>:"Error Cluster From Error Code.vi"("error in (no error)"=w465, "error message (\"\")"="CDB Write/Read fail" ("error message (\"\")"), "error code (0)"=42) -> ("error out"=w464:errorcluster)  [unwired: 6 in]
          }
          frame True {
          }
        }
      }
      frame 200 {
        w513 = T3 2 items=["ANY_HDU"=-1, "IMAGE_HDU"=0, "ASCII_TBL"=1, "BINARY_TBL"=2] ("table type (binary)")
        w483 = "StringV" ("column")
        w514 = T3 1 items=["ANY_HDU"=-1, "IMAGE_HDU"=0, "ASCII_TBL"=1, "BINARY_TBL"=2] ("table type (binary)")
        w506 = "Stringunits" ("units")
        w471 = 2  # row
        w474 = "abcd"  # data
        w485 = "String" ("column")
        n158 = call "gfitsio-open-create-replace-table.vi"("table type (binary)"=w514, "hdu name (dialog if empty)"="ASCII String Data", "error in (no error)"=w518, "gfits refnum"=w519) -> ("error out"=w516:errorcluster, "dup gfits refnum"=w517:T2)  [unwired: 5 in, 1 out]
        n159 = call-poly "gfitsio-write-column.vi"("units"=w506, "row"=w471, "column"=w485, "error in (no error)"=w516, "data"=w474, "gfits refnum"=w517) -> ("error out"=w504:errorcluster, "dup gfits refnum"=w505:T2)  [unwired: 4 in]
        n160 = call "gfitsio-get-current-hdu-info.vi"("error in (no error)"=w504, "gfits refnum"=w505) -> ("error out"=w499:errorcluster, "hdu number"=w497:i32, "dup gfits refnum"=w498:T2)  [unwired: 5 in, 2 out]
        n161 = call "gfitsio-open-create-replace-table.vi"("table type (binary)"=w513, "hdu name (dialog if empty)"="BINARY String Data", "error in (no error)"=w499, "gfits refnum"=w498) -> ("error out"=w508:errorcluster, "dup gfits refnum"=w507:T2)  [unwired: 5 in, 1 out]
        n162 = call-poly "gfitsio-write-column.vi"("units"=w506, "row"=w471, "column"="String", "error in (no error)"=w508, "data"=w474, "Variable Size? (F)"=FALSE ("variable length? (T:yes)"), "gfits refnum"=w507) -> ("error out"=w512:errorcluster, "dup gfits refnum"=w511:T2)  [unwired: 3 in]
        n163 = call-poly "gfitsio-write-column.vi"("units"=w506, "row"=w471, "column"=w483, "error in (no error)"=w512, "data"=w474, "Variable Size? (F)"=TRUE ("variable length? (T:yes)"), "gfits refnum"=w511) -> ("error out"=w503:errorcluster, "dup gfits refnum"=w502:T2)  [unwired: 3 in]
        n164 = call "gfitsio-get-current-hdu-info.vi"("error in (no error)"=w503, "gfits refnum"=w502) -> ("error out"=w501:errorcluster, "hdu number"=w496:i32, "dup gfits refnum"=w500:T2)  [unwired: 5 in, 2 out]
        n165 = call "gfitsio-movabs-hdu.vi"("hdunum"=w497, "error in (no error)"=w501, "gfits refnum"=w500) -> ("error out"=w494:errorcluster, "dup gfits refnum"=w495:T2)  [unwired: 6 in, 1 out]
        n166 = call-poly "gfitsio-read-column.vi"("column"=w485, "error in (no error)"=w494, "row"=w471, "gfits refnum"=w495) -> ("error out"=w490:errorcluster, "data"=w493:string, "dup gfits refnum"=w491:T2)  [unwired: 5 in]
        n167 = Equal?(x=w474, y=w493) -> (x = y?=w482:bool)
        n168 = call "gfitsio-movabs-hdu.vi"("hdunum"=w496, "error in (no error)"=w490, "gfits refnum"=w491) -> ("error out"=w488:errorcluster, "dup gfits refnum"=w489:T2)  [unwired: 6 in, 1 out]
        n169 = call-poly "gfitsio-read-column.vi"("column"=w485, "error in (no error)"=w488, "row"=w471, "gfits refnum"=w489) -> ("error out"=w486:errorcluster, "data"=w492:string, "dup gfits refnum"=w487:T2)  [unwired: 5 in]
        n170 = Equal?(x=w474, y=w492) -> (x = y?=w481:bool)
        n171 = call-poly "gfitsio-read-column.vi"("column"=w483, "error in (no error)"=w486, "row"=w471, "gfits refnum"=w487) -> ("error out"=w478:errorcluster, "data"=w484:string, "dup gfits refnum"=w479:T2)  [unwired: 5 in]
        n172 = Equal?(x=w474, y=w484) -> (x = y?=w480:bool)
        n173 = Compound Arithmetic op=AND(w482, w481, w480) -> (w477:bool)
        n174 = case shown="False" w477 {
          tunnel: w479 -> [w524 w526]
          tunnel: w478 -> [w521 w525]
          tunnel: [w524 w526] -> w476
          tunnel: [w520 w525] -> w475
          frame False {
            n175 = call <vilib>:"Error Cluster From Error Code.vi"("error in (no error)"=w521, "error message (\"\")"="String Write/Read fail" ("error message (\"\")"), "error code (0)"=42) -> ("error out"=w520:errorcluster)  [unwired: 6 in]
          }
          frame True {
          }
        }
      }
      frame 201 {
        w527 = 0.001 ("y")
        w564 = T3 2 items=["ANY_HDU"=-1, "IMAGE_HDU"=0, "ASCII_TBL"=1, "BINARY_TBL"=2] ("table type (binary)")
        w565 = T3 1 items=["ANY_HDU"=-1, "IMAGE_HDU"=0, "ASCII_TBL"=1, "BINARY_TBL"=2] ("table type (binary)")
        w536 = 2  # row
        w537 = timestamp(3446826530.3360677 s since 1904-01-01)  # data
        w543 = "Time" ("column")
        # "Lost in accuracy storing timestamps as strings in FITS file.  Can't test equality here, so check times are within 1ms of each other."
        n176 = call "gfitsio-open-create-replace-table.vi"("table type (binary)"=w565, "hdu name (dialog if empty)"="ASCII Time Data", "error in (no error)"=w569, "gfits refnum"=w570) -> ("error out"=w567:errorcluster, "dup gfits refnum"=w568:T2)  [unwired: 5 in, 1 out]
        n177 = call-poly "gfitsio-write-column.vi"("row"=w536, "column"=w543, "error in (no error)"=w567, "data"=w537, "gfits refnum"=w568) -> ("error out"=w558:errorcluster, "dup gfits refnum"=w559:T2)  [unwired: 5 in]
        n178 = call "gfitsio-get-current-hdu-info.vi"("error in (no error)"=w558, "gfits refnum"=w559) -> ("error out"=w555:errorcluster, "hdu number"=w553:i32, "dup gfits refnum"=w554:T2)  [unwired: 5 in, 2 out]
        n179 = call "gfitsio-open-create-replace-table.vi"("table type (binary)"=w564, "hdu name (dialog if empty)"="BINARY Time Data", "error in (no error)"=w555, "gfits refnum"=w554) -> ("error out"=w561:errorcluster, "dup gfits refnum"=w560:T2)  [unwired: 5 in, 1 out]
        n180 = call-poly "gfitsio-write-column.vi"("row"=w536, "column"="Time", "error in (no error)"=w561, "data"=w537, "gfits refnum"=w560) -> ("error out"=w532:errorcluster, "dup gfits refnum"=w533:T2)  [unwired: 5 in]
        n181 = call "gfitsio-get-current-hdu-info.vi"("error in (no error)"=w532, "gfits refnum"=w533) -> ("error out"=w557:errorcluster, "hdu number"=w552:i32, "dup gfits refnum"=w556:T2)  [unwired: 5 in, 2 out]
        n182 = call "gfitsio-movabs-hdu.vi"("hdunum"=w553, "error in (no error)"=w557, "gfits refnum"=w556) -> ("error out"=w550:errorcluster, "dup gfits refnum"=w551:T2)  [unwired: 6 in, 1 out]
        n183 = call-poly "gfitsio-read-column.vi"("column"=w543, "error in (no error)"=w550, "row"=w536, "gfits refnum"=w551) -> ("error out"=w546:errorcluster, "data"=w549:timestamp, "dup gfits refnum"=w547:T2)  [unwired: 5 in]
        n184 = Subtract(x=w537, y=w549) -> (x-y=w542:dbl)
        n185 = call "gfitsio-movabs-hdu.vi"("hdunum"=w552, "error in (no error)"=w546, "gfits refnum"=w547) -> ("error out"=w544:errorcluster, "dup gfits refnum"=w545:T2)  [unwired: 6 in, 1 out]
        n186 = Absolute Value(x=w542) -> (abs(x)=w531:dbl)
        n187 = call-poly "gfitsio-read-column.vi"("column"=w543, "error in (no error)"=w544, "row"=w536, "gfits refnum"=w545) -> ("error out"=w534:errorcluster, "data"=w548:timestamp, "dup gfits refnum"=w535:T2)  [unwired: 5 in]
        n188 = Subtract(x=w537, y=w548) -> (x-y=w541:dbl)
        n189 = Absolute Value(x=w541) -> (abs(x)=w530:dbl)
        n190 = Less?(x=w531, y=w527) -> (x < y?=w528:bool)
        n191 = Less?(x=w530, y=w527) -> (x < y?=w529:bool)
        n192 = Compound Arithmetic op=AND(w528, w529) -> (w540:bool)
        n193 = case shown="False" w540 {
          tunnel: w535 -> [w575 w577]
          tunnel: w534 -> [w572 w576]
          tunnel: [w575 w577] -> w539
          tunnel: [w571 w576] -> w538
          frame False {
            n194 = call <vilib>:"Error Cluster From Error Code.vi"("error in (no error)"=w572, "error message (\"\")"="Time Write/Read fail" ("error message (\"\")"), "error code (0)"=42) -> ("error out"=w571:errorcluster)  [unwired: 6 in]
          }
          frame True {
          }
        }
      }
      frame 1000 {
      }
    }
  }
  n195 = call "gfitsio-close-file.vi"("error in (no error)"=w1, "gfits refnum"=w2) -> ("error out"=→"error out":errorcluster)  [unwired: 8 in, 1 out]
